vi "Snake.vi"() -> ()   [LabVIEW 2017]
uses:
  Typedef/Snake_states.ctl
panel:
  out "Stop Variable":bool
  out "Score":i32
  out "Snake Field":u32[][](array[colorbox])=[[0, 0, 0, 0, 0, 0, 0, 0, 0, 0, 0, 0, 0, 0, 0, 0, 0, 0, 0, 0, 0, 0, 0, 0, 0, 0, 0], [0, 0, 0, 0, 0, 0, 0, 0, 0, 0, 0, 0, 0, 0, 0, 0, 0, 0, 0, 0, 0, 0, 0, 0, 0, 0, 0], [0, 0, 0, 3622, 0, 0, 0, 0, 0, 0, 0, 0, 0, 0, 0, 0, 0, 0, 0, 0, 0, 0, 0, 0, 0, 0, 0], [0, 0, 0, 0, 0, 0, 0, 0, 0, 0, 0, 0, 0, 0, 0, 0, 0, 0, 0, 0, 0, 0, 0, 0, 0, 0, 0], [0, 0, 0, 0, 0, 0, 0, 0, 0, 0, 0, 0, 0, 0, 0, 0, 0, 0, 0, 0, 0, 0, 0, 0, 0, 0, 0], [0, 0, 0, 0, 0, 0, 0, 0, 0, 0, 0, 0, 0, 0, 0, 0, 0, 0, 0, 0, 0, 0, 0, 0, 0, 0, 0], [0, 0, 0, 0, 0, 0, 0, 0, 0, 0, 0, 0, 0, 0, 0, 0, 0, 0, 0, 0, 0, 0, 0, 0, 0, 0, 0], [0, 0, 0, 0, 0, 0, 0, 0, 0, 0, 0, 0, 0, 0, 0, 0, 0, 0, 0, 0, 0, 0, 0, 0, 0, 0, 0], [0, 0, 0, 0, 0, 0, 0, 0, 0, 0, 0, 0, 0, 0, 0, 0, 0, 0, 0, 0, 0, 0, 0, 0, 0, 0, 0], [0, 0, 0, 0, 0, 0, 0, 0, 0, 0, 0, 0, 0, 0, 0, 0, 0, 0, 0, 0, 0, 0, 0, 0, 0, 0, 0], [0, 0, 0, 0, 0, 0, 0, 0, 0, 0, 0, 0, 0, 0, 0, 0, 0, 0, 0, 0, 0, 0, 0, 0, 0, 0, 0], [0, 0, 0, 0, 0, 0, 0, 0, 0, 0, 0, 0, 0, 0, 0, 0, 0, 0, 0, 0, 0, 0, 0, 0, 0, 0, 0], [0, 0, 0, 0, 0, 0, 0, 0, 0, 0, 0, 0, 0, 0, 0, 0, 0, 0, 0, 0, 0, 0, 0, 0, 0, 0, 0], [0, 0, 0, 0, 0, 0, 0, 0, 0, 0, 0, 0, 0, 0, 0, 0, 0, 0, 0, 0, 0, 0, 0, 0, 0, 0, 0], [0, 0, 0, 0, 0, 0, 0, 0, 0, 0, 0, 0, 0, 0, 0, 0, 0, 0, 0, 0, 0, 0, 0, 0, 0, 0, 0], [0, 0, 0, 0, 0, 0, 0, 0, 0, 0, 0, 0, 0, 0, 0, 0, 0, 0, 0, 0, 0, 0, 0, 0, 0, 0, 0], [0, 0, 0, 0, 0, 0, 0, 0, 0, 0, 0, 0, 0, 0, 0, 0, 0, 0, 0, 0, 0, 0, 0, 0, 0, 0, 0], [0, 0, 0, 0, 0, 0, 0, 0, 0, 0, 0, 0, 0, 0, 0, 0, 0, 0, 0, 0, 0, 0, 0, 0, 0, 0, 0], [0, 0, 0, 0, 0, 0, 0, 0, 0, 0, 0, 0, 0, 0, 0, 0, 0, 0, 0, 0, 0, 0, 0, 0, 0, 0, 0], [0, 0, 0, 0, 0, 0, 0, 0, 0, 0, 0, 0, 0, 0, 0, 0, 0, 0, 0, 0, 0, 0, 0, 0, 0, 0, 0]]
  out "Y Direction":i32
  out "X Direction":i32
  in  "Stop":bool
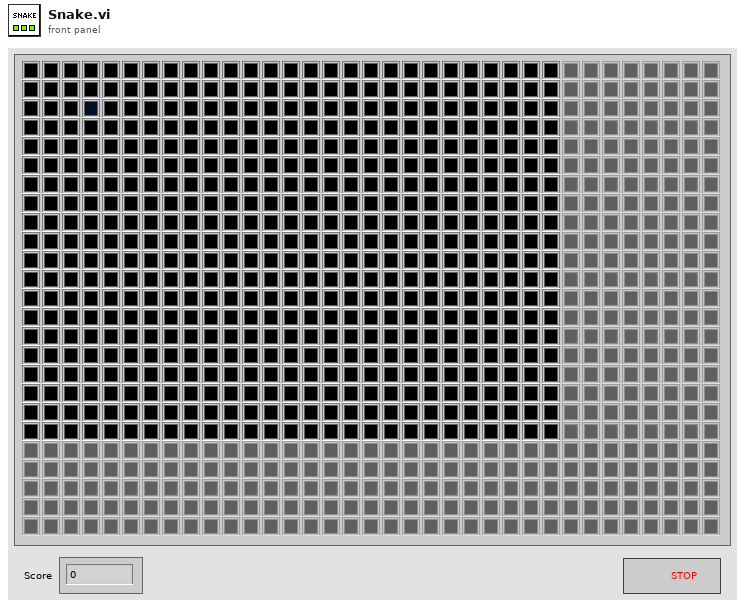
[diagram p1: front panel]
types:
  T1 = typedef "Snake_states.ctl" = enum16{"Initialize", "Start game", "Wait for user to press button", "Stop"}
  T2 = typedef "eventvkey.ctl" = enum16{"ASCII", "Enter", "Return", "Shift", "Ctrl", "Alt", "Cmd", "Opt", "Caps", "NumLock", "Clear", "Break", "Up", "Down", "Left", "Right", "Insert", "Delete", "Home", "End", "PageUp", "PageDown", "Escape", "Help", "Pause", "ScrollLock", "F1", "F2", "F3", "F4", "F5", "F6", "F7", "F8", "F9", "F10", "F11", "F12", "F13", "F14", "F15", "F16", "F17", "F18", "F19", "F20", "F21", "F22", "F23", "F24", "Play", "VolumeUp", "VolumeDown", "Mute", "Two Byte Char"}
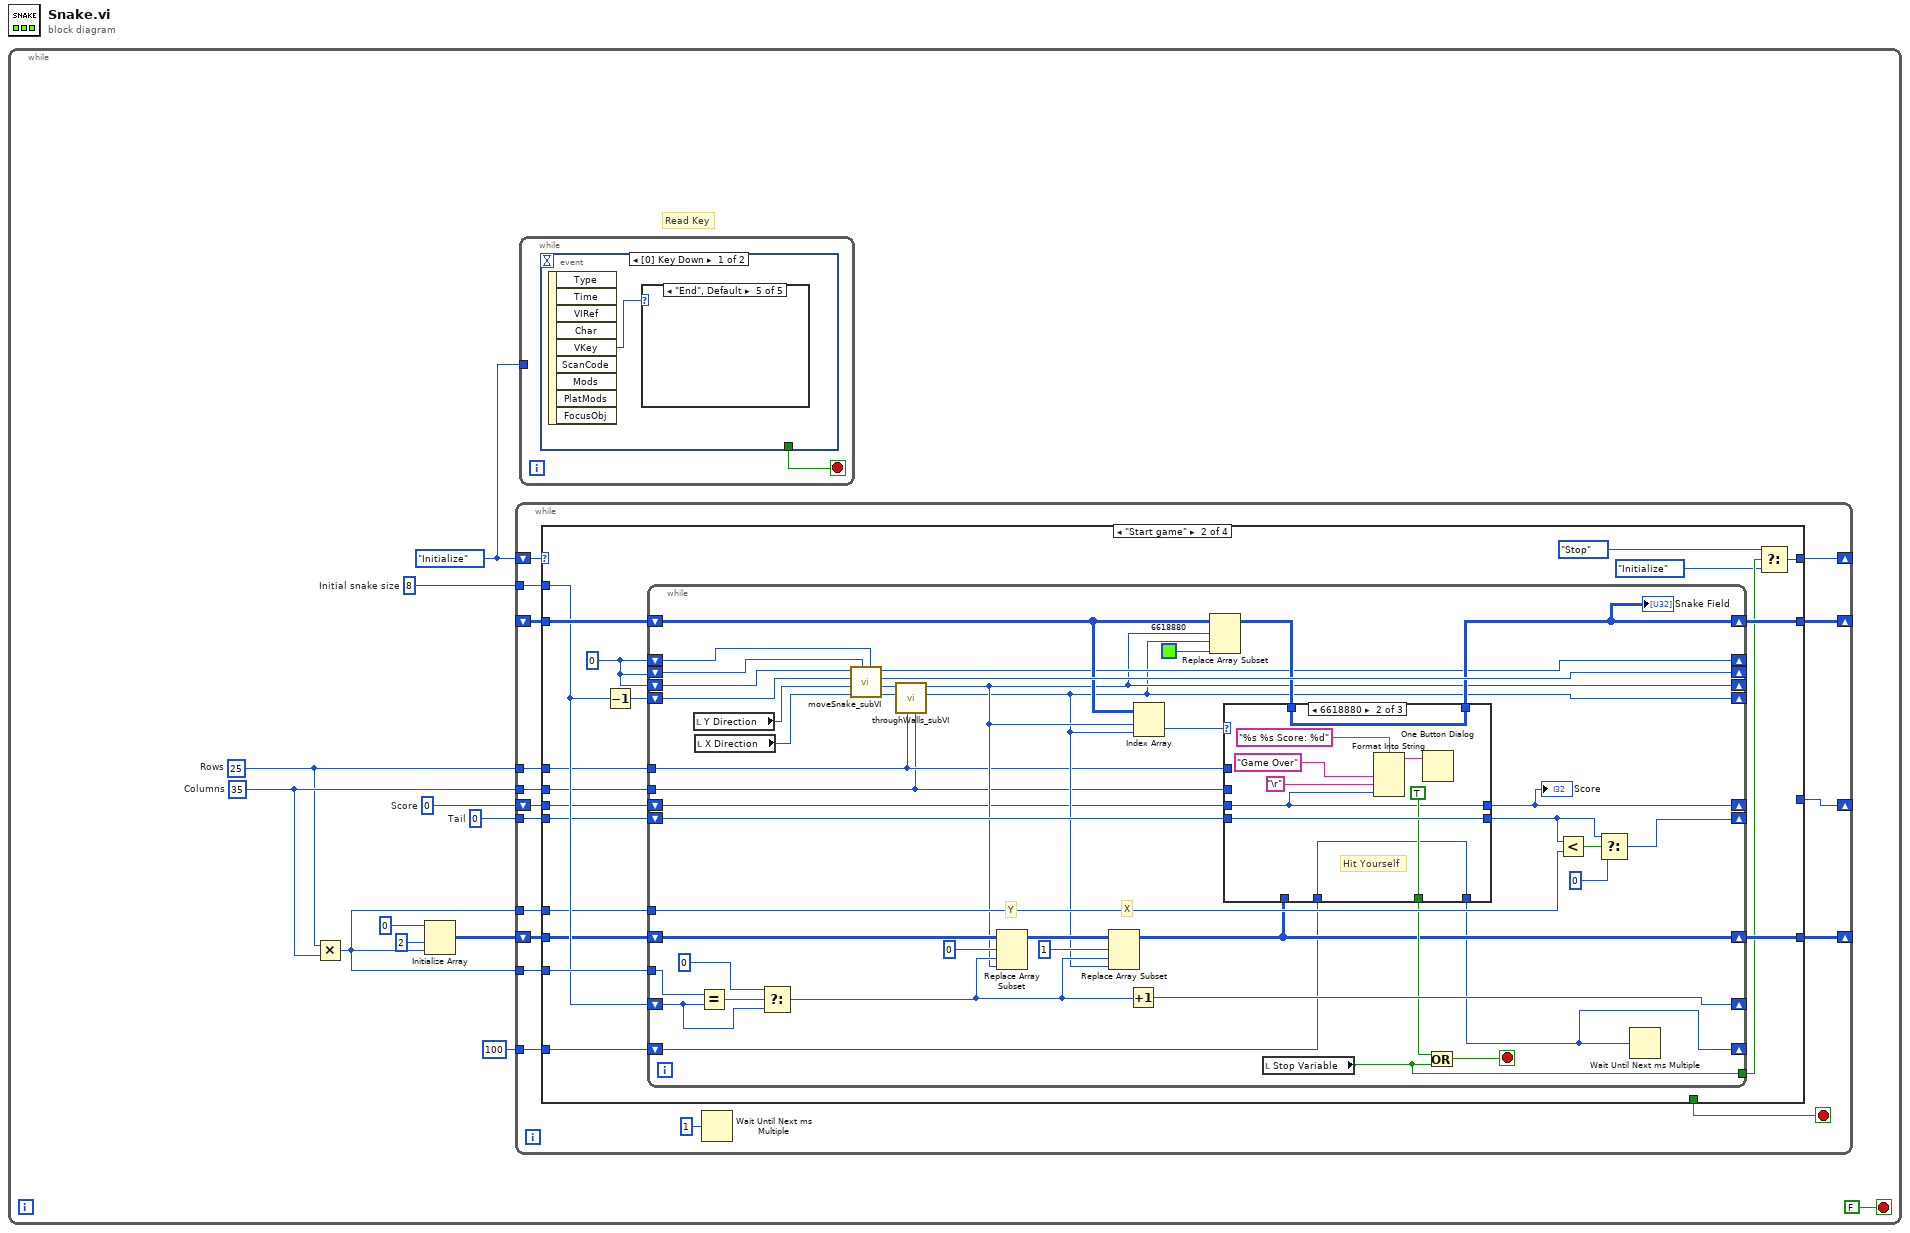
[diagram p0: block diagram]
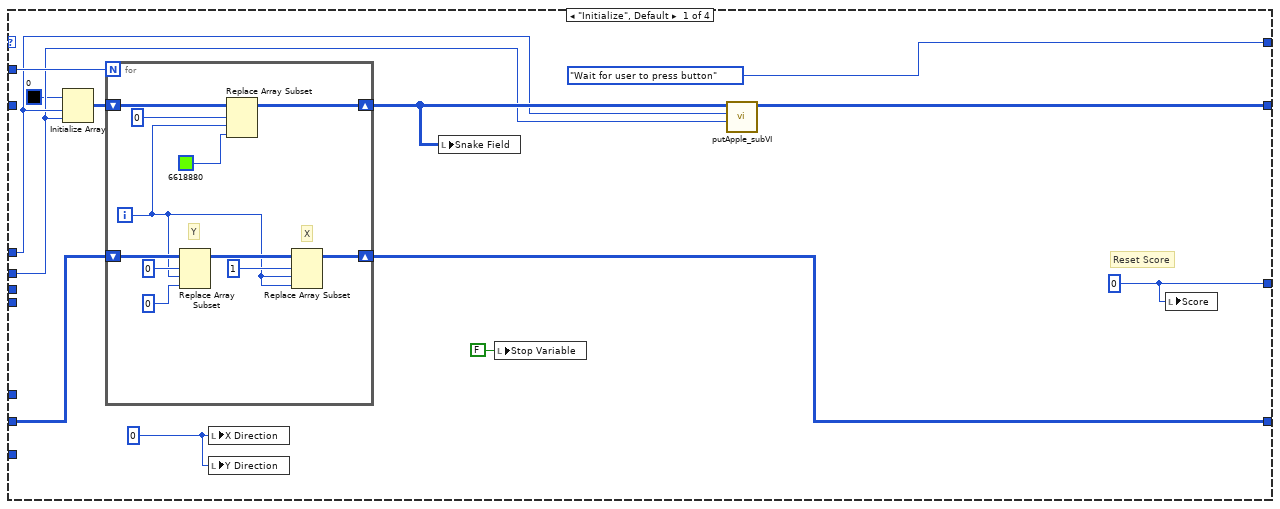
[diagram p2: hidden frame]
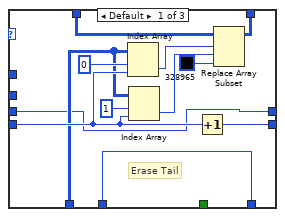
[diagram p3: hidden frame]
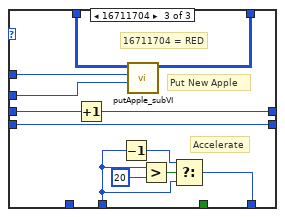
[diagram p4: hidden frame]
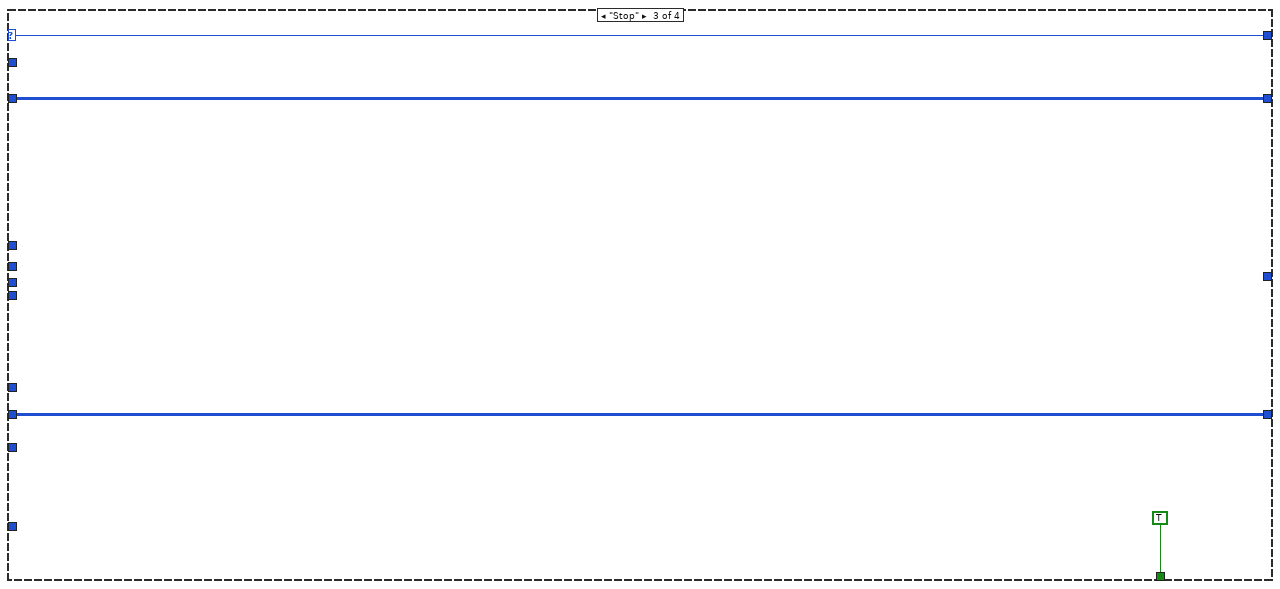
[diagram p5: hidden frame]
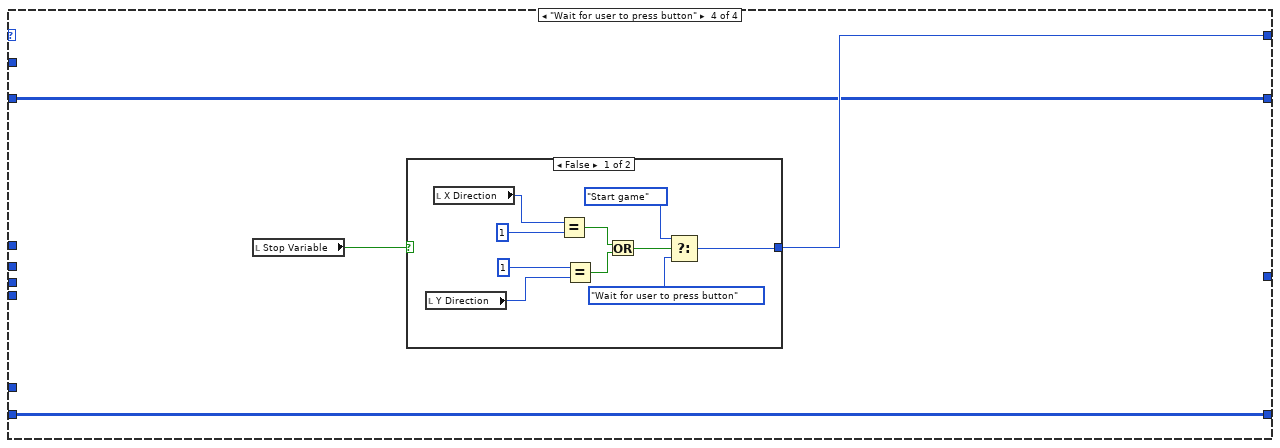
[diagram p6: hidden frame]
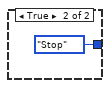
[diagram p7: hidden frame]
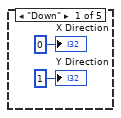
[diagram p8: hidden frame]
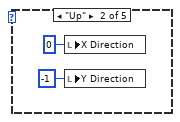
[diagram p9: hidden frame]
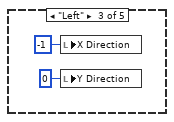
[diagram p10: hidden frame]
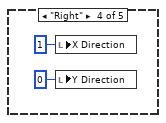
[diagram p11: hidden frame]
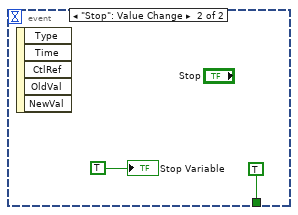
[diagram p12: hidden frame]
diagram:
  n1 = while {
    stop <- FALSE stop-if-true
    w3 = 0  # Score
    w7 = 0  # Tail
    w11 = 8  # Initial snake size
    w6 = 35  # Columns
    w5 = 25  # Rows
    w12 = Snake_states."Initialize"
    # "Read Key"
    n2 = Multiply(x=w5, y=w6) -> (x*y=w4:i32)
    n3 = Initialize Array(0 ("element"), 2 ("dimension size"), w4) -> (w8:i32[][])
    n4 = while {
      shift-right: [w28] -> _
      shift-left: w12 -> [w29]
      tunnel: w4 -> [w26]
      tunnel: w11 -> [w25]
      shift-right: [w24] -> _
      shift-left: _ -> [w27]
      shift-right: [w22] -> _
      shift-left: w8 -> [w23]
      tunnel: w7 -> [w21]
      tunnel: w6 -> [w20]
      tunnel: w5 -> [w19]
      tunnel: w4 -> [w18]
      shift-right: [w15] -> _
      shift-left: w3 -> [w16]
      tunnel: u32 100 ("Speed") -> [w14]
      stop <- w17 stop-if-true
      n5 = case shown="\"Start game\"" w29 {
        selector: w29 -> [_ _ w151 _]
        tunnel: [Snake_states."Wait for user to press button" w60 w151 w155] -> w28
        tunnel: w27 -> [_ w71 w150 w154]
        tunnel: w26 -> [_ w70 _ _]
        tunnel: w25 -> [w40 w67 _ _]
        tunnel: [w36 w69 w150 w154] -> w24
        tunnel: w23 -> [w39 w66 w149 w153]
        tunnel: [w38 w65 w149 w153] -> w22
        tunnel: w19 -> [w35 w64 _ _]
        tunnel: w20 -> [w34 w63 _ _]
        tunnel: w21 -> [_ w62 _ _]
        tunnel: w18 -> [_ w61 _ _]
        tunnel: [_ _ TRUE _] -> w17
        tunnel: w16 -> [_ w55 _ _]
        tunnel: [w31 _ _ _] -> w15
        tunnel: w14 -> [_ w54 _ _]
        frame "Initialize", Default {
          w31 = 0 ("index (row)")
          w41 = 0 ("X Direction")
          # "Reset Score"
          n6 = Initialize Array(u32 0 ("Color Box"), w35, w34) -> (w32:u32[][])
          n7 = for {
            N: w40 -> [_]
            shift-right: [w50] -> w37
            shift-left: w32 -> [w52]
            shift-right: [w43] -> w38
            shift-left: w39 -> [w48]
            i -> [w44]
            # "X"
            # "Y"
            n8 = Replace Array Subset(array=w48, new element=0 ("new element/subarray"), index (row)=0, index (col)=w44) -> (w47:i32[][])
            n9 = Replace Array Subset(array=w52, new element=u32 6618880 ("Color Box"), index (row)=0, index (col)=w44) -> (w50:u32[][])
            n10 = Replace Array Subset(array=w47, new element=w44, index (row)=1, index (col)=w44) -> (w43:i32[][])
          }
          n11 = local write "X Direction"(w41) -> ()
          n12 = local write "Y Direction"(w41) -> ()
          n13 = local write "Snake Field"(w37) -> ()
          n14 = local write "Stop Variable"(FALSE ("Stop Variable")) -> ()
          n15 = call "putApple_subVI.vi"("Field Width"=w34, "Field Height"=w35, "Snake Field in"=w37) -> ("Snake Field out"=w36:u32[][])  [unwired: 8 in]
          n16 = local write "Score"(w31) -> ()
        }
        frame "Start game" {
          w56 = 0 ("Current Direction Y")
          n17 = Decrement(x=w67) -> (x-1=w68:i32)
          n18 = while {
            shift-right: [w81] -> _
            shift-left: w56 -> [w114]
            shift-right: [w80] -> _
            shift-left: w68 -> [w113]
            shift-right: [w95] -> w69
            shift-left: w71 -> [w94]
            tunnel: w70 -> [w108]
            shift-right: [w109] -> _
            shift-left: w67 -> [w105]
            shift-right: [w77] -> w65
            shift-left: w66 -> [w104]
            tunnel: w64 -> [w79]
            tunnel: w63 -> [w78]
            shift-right: [w84] -> _
            shift-left: w56 -> [w98]
            shift-right: [w99] -> _
            shift-left: w56 -> [w97]
            shift-right: [w88] -> _
            shift-left: w62 -> [w93]
            tunnel: w61 -> [w92]
            tunnel: [w72] -> w59
            shift-right: [w75] -> _
            shift-left: w55 -> [w76]
            shift-right: [w73] -> _
            shift-left: w54 -> [w74]
            stop <- w86 stop-if-true
            # "X"
            # "Y"
            n19 = local read "Y Direction"() -> (w112:i32)
            n20 = local read "X Direction"() -> (w111:i32)
            n21 = Equal?(x=w108, y=w105) -> (x = y?=w107:bool)
            n22 = Select(t=0, s=w107, f=w105) -> (s? t:f=w100:i32)
            n23 = call "moveSnake_subVI.vi"("Old Direction Y"=w98, "Old Direction X"=w97, "New Direction X"=w111, "New Direction Y"=w112, "Snake Head X"=w113, "Snake Head Y"=w114) -> ("New Snake Head X"=w82:i32, "New Snake Head Y"=w83:i32, "Current Direction X"=w99:i32, "Current Direction Y"=w84:i32)  [unwired: 2 in]
            n24 = call "throughWalls_subVI.vi"("Columns"=w78, "Rows"=w79, "Next X"=w82, "Next Y"=w83) -> ("Next X"=w80:i32, "Next Y"=w81:i32)  [unwired: 6 in]
            n25 = Replace Array Subset(array=w104, new element=w81, index (row)=0, index (col)=w100) -> (w103:i32[][])
            n26 = Replace Array Subset(array=w103, new element=w80, index (row)=1, index (col)=w100) -> (w77:i32[][])
            n27 = Increment(x=w100) -> (x+1=w109:i32)
            n28 = Index Array(array=w94, index (row)=w81, index (col)=w80) -> (element=w87:u32)
            n29 = Replace Array Subset(array=w94, new element=u32 6618880 ("Color Box"), index (row)=w81, index (col)=w80) -> (w96:u32[][])
            n30 = case shown="6618880" w87 {
              tunnel: w79 -> [_ _ w146]
              tunnel: w78 -> [_ _ w145]
              tunnel: w96 -> [w126 w135 w147]
              tunnel: [w125 w135 w144] -> w95
              tunnel: w93 -> [w119 w134 w143]
              tunnel: [w118 w134 w143] -> w90
              tunnel: [_ TRUE _] -> w85
              tunnel: w77 -> [w117 _ _]
              tunnel: w76 -> [w116 w129 w142]
              tunnel: [w116 w129 w141] -> w75
              tunnel: w74 -> [w115 w127 w136]
              tunnel: [w115 w127 w137] -> w73
              frame Default {
                # "Erase Tail"
                n31 = Index Array(array=w117, index (row)=0 ("disabled index (row)"), index (col)=w119) -> (element=w120:i32)
                n32 = Index Array(array=w117, index (row)=1, index (col)=w119) -> (element=w123:i32)
                n33 = Increment(x=w119) -> (x+1=w118:i32)
                n34 = Replace Array Subset(array=w126, new element=u32 328965 ("Color Box"), index (row)=w120, index (col)=w123) -> (w125:u32[][])
              }
              frame 6618880 {
                # "Hit Yourself"
                n35 = Format Into String(format string="%s %s Score: %d", "Game Over", "\r", w129) -> (resulting string=w130:string)  [unwired: 2 in, 1 out]
                n36 = One Button Dialog(message=w130) -> ()  [unwired: 1 in, 1 out]
              }
              frame 16711704 {
                # "Accelerate"
                # "16711704 = RED"
                # "Put New Apple"
                n37 = Increment(x=w142) -> (x+1=w141:i32)
                n38 = Decrement(x=w136) -> (x-1=w138:u32)
                n39 = call "putApple_subVI.vi"("Field Width"=w145, "Field Height"=w146, "Snake Field in"=w147) -> ("Snake Field out"=w144:u32[][])  [unwired: 8 in]
                n40 = Greater?(x=w136, y=u32 20) -> (0:w139:bool)
                n41 = Select(t=w138, s=w139, f=w136) -> (s? t:f=w137:u32)
              }
            }
            "Snake Field" <- w95
            "Score" <- w75
            n42 = local read "Stop Variable"() -> (w72:bool)
            n43 = Or(x=w85, y=w72) -> (x .or. y?=w86:bool)
            n44 = Less?(x=w90, y=w92) -> (x < y?=w91:bool)
            n45 = Select(t=w90, s=w91, f=0) -> (s? t:f=w88:i32)
            n46 = Wait Until Next ms Multiple(millisecond multiple=w73) -> ()  [unwired: 1 out]
          }
          n47 = Select(t=Snake_states."Stop", s=w59, f=Snake_states."Initialize") -> (s? t:f=w60:T1)
        }
        frame "Stop" {
        }
        frame "Wait for user to press button" {
          n48 = local read "Stop Variable"() -> (w152:bool)
          n49 = case shown="False" w152 {
            tunnel: [w156 Snake_states."Stop"] -> w155
            frame False {
              n50 = local read "Y Direction"() -> (w165:i32)
              n51 = local read "X Direction"() -> (w163:i32)
              n52 = Equal?(x=w163, y=1) -> (x = y?=w160:bool)
              n53 = Equal?(x=1, y=w165) -> (x = y?=w161:bool)
              n54 = Or(x=w160, y=w161) -> (x .or. y?=w159:bool)
              n55 = Select(t=Snake_states."Start game", s=w159, f=Snake_states."Wait for user to press button") -> (s? t:f=w156:T1)
            }
            frame True {
            }
          }
        }
      }
      n56 = Wait Until Next ms Multiple(millisecond multiple=u32 1) -> ()  [unwired: 1 out]
    }
    n57 = while {
      tunnel: w12 -> [_]
      stop <- w167 stop-if-true
      n58 = event shown="[0] Key Down" {
        selector: _ -> [_ _]
        dyn-events: _ -> [_ _]
        timeout: _ -> [_ _]
        tunnel: [_ TRUE] -> w167
        event Key Down {
          n59 = event-data() -> ("VKey"=w168:T2)  [unwired: 1 in, 8 out]
          n60 = case shown="\"End\", Default" w168 {
            frame "Down" {
              "X Direction" <- 0 ("X Direction")
              "Y Direction" <- 1 ("Y Direction")
            }
            frame "Up" {
              n61 = local write "X Direction"(0 ("X Direction")) -> ()
              n62 = local write "Y Direction"(-1 ("Y Direction")) -> ()
            }
            frame "Left" {
              n63 = local write "X Direction"(-1 ("X Direction")) -> ()
              n64 = local write "Y Direction"(0 ("Y Direction")) -> ()
            }
            frame "Right" {
              n65 = local write "X Direction"(1 ("X Direction")) -> ()
              n66 = local write "Y Direction"(0 ("Y Direction")) -> ()
            }
            frame "End", Default {
            }
          }
        }
        event "Stop": Value Change {
          n67 = event-data() -> ()  [unwired: 1 in, 5 out]
          "Stop Variable" <- TRUE
        }
      }
    }
  }
